vi "deltaHRT.vi"(9 "data input":T3, 10 "Coagulant":T1={"flocculator volume (L)"=100.0, "clarifier volume (L)"=0.0, "dose updates per HRT"=0, "target clarified turbidity (NTU)"=0.3, "Coagulant mode"=enum."Manual", "Coag dose [mg/L]"=0.0} {"target clarified turbidity (NTU)" min=0.1 max=5.0 step=0.01; "dose updates per HRT" min=1 max=1000 step=1}, 11 "seconds since 1Jan1904":timestamp) -> (1 "new interval":bool, 2 "sum HRT":dbl, 3 "total HRT":dbl)   [LabVIEW 2015]
uses:
  coag.ctl
  Manual or Auto.ctl
panel:
  out "delta HRT":dbl
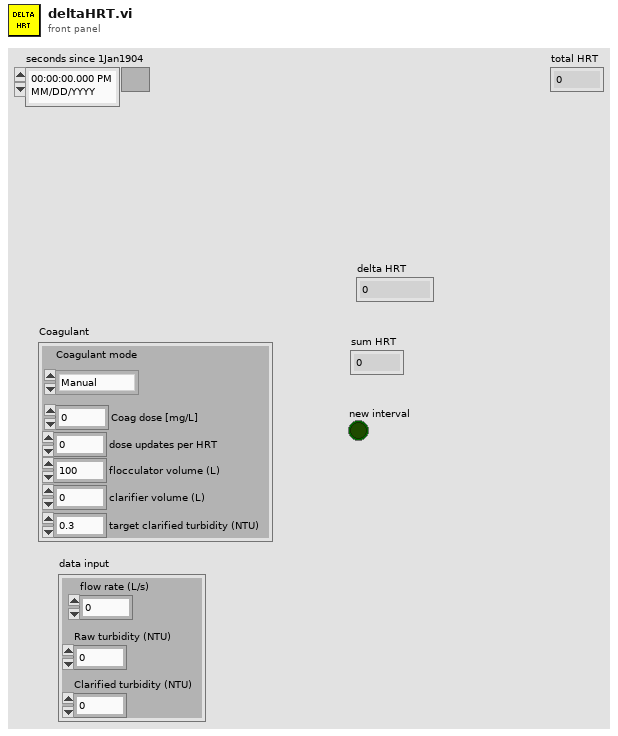
[diagram p1: front panel]
types:
  T1 = typedef "coag.ctl" = cluster{"flocculator volume (L)":dbl, "clarifier volume (L)":dbl, "dose updates per HRT":u32, "target clarified turbidity (NTU)":dbl, "Coagulant mode":T2, "Coag dose [mg/L]":dbl}
  T2 = typedef "Manual or Auto.ctl" = enum16{"Manual", "Automatic"}
  T3 = cluster{"Clarified turbidity (NTU)":dbl, "Raw turbidity (NTU)":dbl, "flow rate (L/s)":dbl}
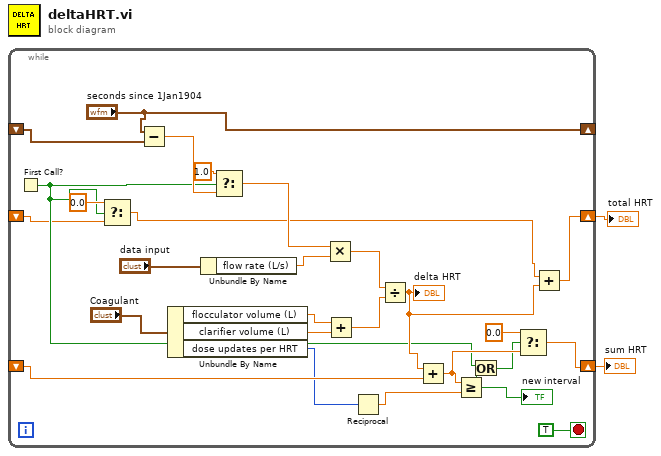
[diagram p0: block diagram]
diagram:
  n1 = while {
    shift-right: ["seconds since 1Jan1904"] -> _
    shift-left: _ -> [w21]
    shift-right: [w14] -> w2
    shift-left: _ -> [w15]
    shift-right: [w8] -> w1
    shift-left: _ -> [w4]
    stop <- TRUE stop-if-true
    n2 = First Call?() -> (First Call?: T/F=w5:bool)
    n3 = Select(t=0.0, s=w5, f=w4) -> (s? t:f=w3:dbl)
    n4 = Subtract(x="seconds since 1Jan1904", y=w21) -> (x-y=w19:dbl)
    n5 = Unbundle By Name("Coagulant") -> ("flocculator volume (L)"=w26:dbl, "clarifier volume (L)"=w25:dbl, "dose updates per HRT"=w10:u32)
    n6 = Unbundle By Name("data input") -> ("flow rate (L/s)"=w27:dbl)
    n7 = Select(t=1.0, s=w5, f=w19) -> (s? t:f=w17:dbl)
    n8 = Multiply(x=w17, y=w27) -> (x*y=w24:dbl)
    n9 = Add(x=w26, y=w25) -> (x+y=w23:dbl)
    n10 = Reciprocal(x=w10) -> (1/x=w9:dbl)
    n11 = Divide(x=w24, y=w23) -> (x/y=w7:dbl)
    "delta HRT" <- w7
    n12 = Add(x=w7, y=w15) -> (x+y=w12:dbl)
    n13 = Greater Or Equal?(x=w12, y=w9) -> (x >= y?=w13:bool)
    "new interval" <- w13
    n14 = Or(x=w5, y=w13) -> (x .or. y?=w11:bool)
    n15 = Select(t=0.0, s=w11, f=w12) -> (s? t:f=w14:dbl)
    n16 = Add(x=w3, y=w7) -> (x+y=w8:dbl)
  }
  "sum HRT" <- w2
  "total HRT" <- w1
